vi "Subtract DAQ Offset.vi"(8 "error in (no error)":errorcluster, 9 "DAQ Offset":dbl[](array[numeric]), 10 "WFM in":waveform(dbl)[](array[waveform]), 11 "Lockin.DAQ":refnum<class "Lockin.DAQ.lvclass">) -> (0 "error out":errorcluster, 2 "WFM out":waveform(dbl)[](array[waveform]), 3 "Lockin.DAQ out":refnum<class "Lockin.DAQ.lvclass">)   [LabVIEW 2016, in "Lockin.DAQ.lvclass"]
uses:
  Lockin.DAQ.lvclass
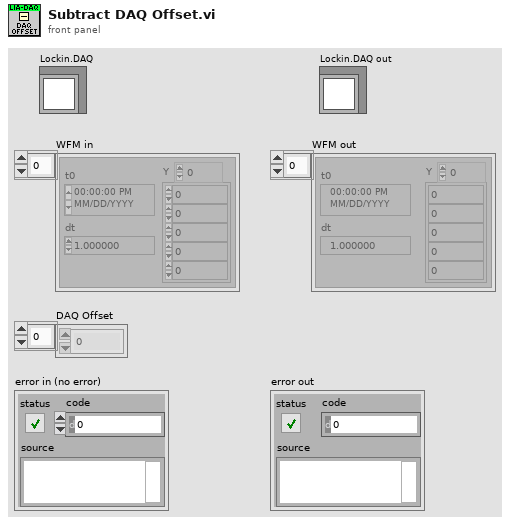
[diagram p1: front panel]
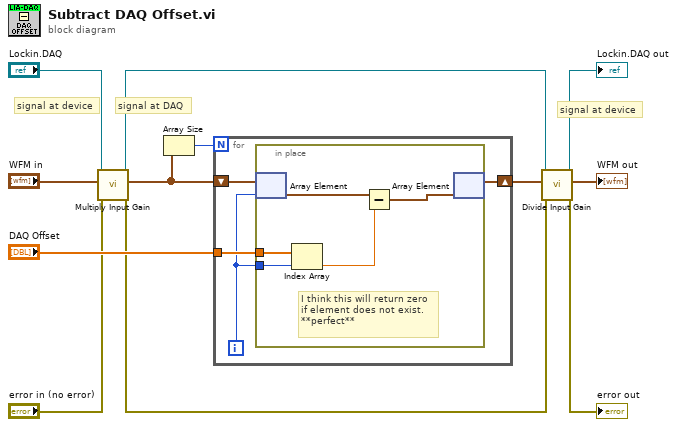
[diagram p0: block diagram]
diagram:
  # "signal at device"
  # "signal at DAQ"
  # "signal at device"
  n1 = call "Multiply Input Gain.vi"("error in (no error)"="error in (no error)", "WFM in"="WFM in", "Lockin.DAQ"="Lockin.DAQ") -> ("error out"=w3:errorcluster, "WFM out"=w9:waveform(dbl)[], "Lockin.DAQ out"=w2:refnum<class "Lockin.DAQ.lvclass">)  [unwired: 6 in]
  n2 = Array Size(array=w9) -> (size(s)=w11:i32)
  n3 = for {
    N: w11 -> [_]
    tunnel: "DAQ Offset" -> [w16]
    shift-right: [w13] -> w7
    shift-left: w9 -> [w14]
    i -> [w15]
    n4 = in-place {
      in-place-border: w15 -> [w21]
      in-place-border: w16 -> [w20]
      # "I think this will return zero\nif element does not exist.\n**perfect**"
      n5 = in-place-array #1(w14, w15) -> (w17:waveform(dbl))
      n6 = Index Array(array=w20, index=w21) -> (element=w19:dbl)
      n7 = Subtract(x=w17, y=w19) -> (x-y=w18:waveform(dbl))
      n8 = in-place-array #1(w18) -> (w13:waveform(dbl)[])  [unwired: 1 out]
    }
  }
  n9 = call "Divide Input Gain.vi"("error in (no error)"=w3, "WFM in"=w7, "Lockin.DAQ"=w2) -> ("error out"=→"error out":errorcluster, "WFM out"=→"WFM out":waveform(dbl)[], "Lockin.DAQ out"=→"Lockin.DAQ out":refnum<class "Lockin.DAQ.lvclass">)  [unwired: 6 in]
